vi "Compress Message Data.vi"(11 "Message":string) -> (3 "Compressed Message":u8[](array[numeric]))   [LabVIEW 2020]
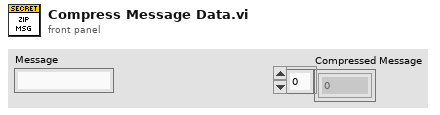
[diagram p1: front panel]
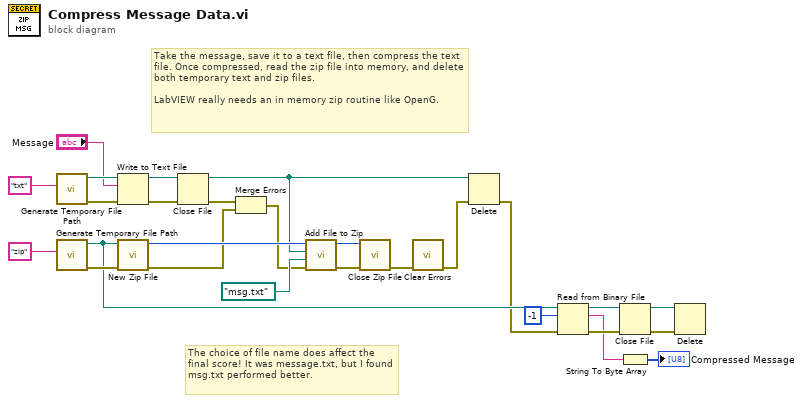
[diagram p0: block diagram]
diagram:
  # "The choice of file name does affect the final score! It was message.txt, but I found msg.txt performed better."
  # "Take the message, save it to a text file, then compress the text file. Once compressed, read the zip file into memory, and delete both temporary text and zip files.\n\nLabVIEW really needs an in memory zip routine like OpenG."
  n1 = call <vilib>:"Generate Temporary File Path.vi"("Temporary File Extension (tmp)"="txt") -> ("error out"=w19:errorcluster, "Unique Temporary File Path"=w27:path)  [unwired: 9 in]
  n2 = call <vilib>:"Generate Temporary File Path.vi"("Temporary File Extension (tmp)"="zip") -> ("error out"=w18:errorcluster, "Unique Temporary File Path"=w10:path)  [unwired: 9 in]
  n3 = Write to Text File(file (use dialog)=w27, text="Message", error in=w19) -> (refnum out=w23:refnum<file>, error out=w17:errorcluster)  [unwired: 1 in, 1 out]
  n4 = call <vilib>:"New Zip File.vi"("error in (no error)"=w18, "target"=w10) -> ("error out"=w16:errorcluster, "zip file out"=w25:i64)  [unwired: 3 in, 1 out]
  n5 = Close File(refnum=w23, error in=w17) -> (path=w13:path, error out=w14:errorcluster)
  n6 = Merge Errors(w14, w16) -> (w15:errorcluster)
  n7 = call <vilib>:"Add File to Zip.vi"("error in (no error)"=w15, "destination path in zip"=path "msg.txt", "source file path"=w13, "zip file in"=w25) -> ("error out"=w20:errorcluster, "zip file out"=w21:i64)  [unwired: 6 in]
  n8 = call <vilib>:"Close Zip File.vi"("error in (no error)"=w20, "zip file in"=w21) -> ("error out"=w12:errorcluster)  [unwired: 5 in]
  n9 = call <vilib>:"Clear Errors.vi"("error in (no error)"=w12) -> ("error out"=w11:errorcluster)  [unwired: 5 in, 1 out]
  n10 = Delete(path (use dialog)=w13, error in=w11) -> (error out=w9:errorcluster)  [unwired: 3 in, 2 out]
  n11 = Read from Binary File(8:w9, 10:-1 ("count (1)"), 11:w10) -> (0:w6:errorcluster, 2:w2:string, 3:w7:refnum<file>)  [unwired: 3 in, 1 out]
  n12 = Close File(refnum=w7, error in=w6) -> (path=w5:path, error out=w4:errorcluster)
  n13 = String To Byte Array(string=w2) -> (unsigned byte array=→"Compressed Message":u8[])
  n14 = Delete(path (use dialog)=w5, error in=w4) -> ()  [unwired: 3 in, 3 out]
